vi "Default Variant.vi"(1 "type code":T1) -> (0 "Variant":variant)   [LabVIEW 2020, in "Value.lvlib"]
uses:
  Value.lvlib
  Type Code.ctl
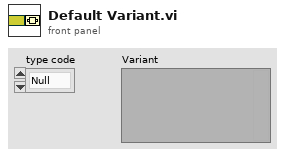
[diagram p1: front panel]
types:
  T1 = typedef "Value.lvlib/Type Code.ctl" = enum8{"Null", "Bool", "BoolA", "Int8", "Int8A", "Int16", "Int16A", "Int32", "Int32A", "Int64", "Int64A", "UInt8", "UInt8A", "UInt16", "UInt16A", "UInt32", "UInt32A", "UInt64", "UInt64A", "Float32", "Float32A", "Float64", "Float64A", "String", "StringA", "Struct", "StructA", "Union", "UnionA", "Any", "AnyA"}
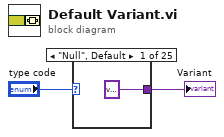
[diagram p0: block diagram]
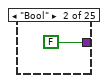
[diagram p2: hidden frame]
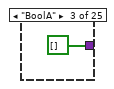
[diagram p3: hidden frame]
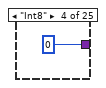
[diagram p4: hidden frame]
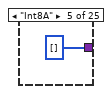
[diagram p5: hidden frame]
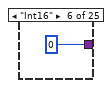
[diagram p6: hidden frame]
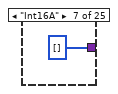
[diagram p7: hidden frame]
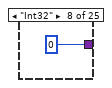
[diagram p8: hidden frame]
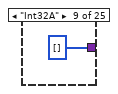
[diagram p9: hidden frame]
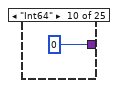
[diagram p10: hidden frame]
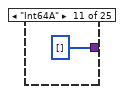
[diagram p11: hidden frame]
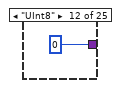
[diagram p12: hidden frame]
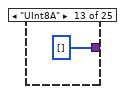
[diagram p13: hidden frame]
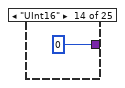
[diagram p14: hidden frame]
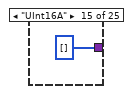
[diagram p15: hidden frame]
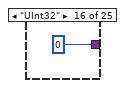
[diagram p16: hidden frame]
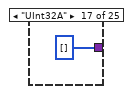
[diagram p17: hidden frame]
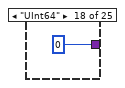
[diagram p18: hidden frame]
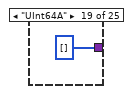
[diagram p19: hidden frame]
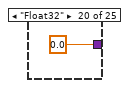
[diagram p20: hidden frame]
diagram:
  n1 = case shown="\"Null\", Default" "type code" {
    tunnel: [variant FALSE bool[] [] i8 0 i8[] [] i16 0 i16[] [] 0 i32[] [] i64 0 i64[] [] u8 0 u8[] [] u16 0 u16[] [] u32 0 u32[] [] u64 0 u64[] [] sgl 0.0 0.0 sgl[] [] dbl[] [] "" string[] []] -> w1
    frame "Null", Default {
    }
    frame "Bool" {
    }
    frame "BoolA" {
    }
    frame "Int8" {
    }
    frame "Int8A" {
    }
    frame "Int16" {
    }
    frame "Int16A" {
    }
    frame "Int32" {
    }
    frame "Int32A" {
    }
    frame "Int64" {
    }
    frame "Int64A" {
    }
    frame "UInt8" {
    }
    frame "UInt8A" {
    }
    frame "UInt16" {
    }
    frame "UInt16A" {
    }
    frame "UInt32" {
    }
    frame "UInt32A" {
    }
    frame "UInt64" {
    }
    frame "UInt64A" {
    }
    frame "Float32" {
    }
    frame "Float64" {
    }
    frame "Float32A" {
    }
    frame "Float64A" {
    }
    frame "String" {
    }
    frame "StringA" {
    }
  }
  "Variant" <- w1
